vi "Constants.vi"() -> ()   [LabVIEW 2015, in "DDS Custom Device Shared.lvlib"]
doc: "Use this Global VI to access the GUIDs assigned to the page resources of the Custom Device."
uses:
  DDS Custom Device Shared.lvlib
panel:
  in  "Tab Control":enum32{"GUIDS", "Constants", "Properties"}(tab)=enum."Properties"
  in  "GUID Writer Channel":string="796baeca-3510-460a-ac62-f01a5eb8fe3f"
  in  "GUID Reader Page":string="796baeca-3510-460a-ac62-f01a5eb8fe3f"
  in  "GUID Readers Section":string="6c820a71-c73a-43d9-b216-f9ee8b776095"
  in  "GUID Writer Page":string="79fac92f-d032-46dc-bd23-f82c2cfdfdbc"
  in  "GUID Writers Section":string="dd125e97-1a18-47b4-aa06-ca880e6dc00e"
  in  "GUID DDS Custom Device":string="e2ce4079-becb-402d-aff2-142c98505f69"
  in  "Topic Cluster Bool Channel Name":string="Cluster_Bool"
  in  "Topic Cluster Sgl_Num Channel Name":string="Cluster_Sgl_Num"
  in  "Topic Sgl_Array Channel Name":string="Sgl_Array_Elem"
  in  "Topic U16_Num Channel Name":string="U16_Num"
  in  "Topic I64_Num Channel Name":string="I64_Num"
  in  "Topic I32_Num Channel Name":string="I32_Num"
  in  "Readers Section Name":string="Topic Readers"
  in  "Topic Name":string="MyTopic"
  in  "Writers Section Name":string="Topic Writers"
  in  "Channel.DataType":string="U32"
  in  "Topic.forceRead":string="forceRead"
  in  "Topic.forceExclusiveReader":string="forceExclusiveReader"
  in  "Topic.keyName":string="keyName"
  in  "Topic.forceUnboundedString":string="forceUnboundedString"
  in  "Topic.forceArrayMapping":string="forceArrayMapping"
  in  "Topic.dataWriterParticipantQoSProfile":string="dataWriterQoS"
  in  "Topic.domainParticipantQoSProfile":string="participantQoS"
  in  "Topic.typeName":string="typeName"
  in  "Topic.topicName":string="topicWriterName"
  in  "Topic.domainId":string="domainId"
  in  "Compiled.Settings":string="Compiled.Settings"
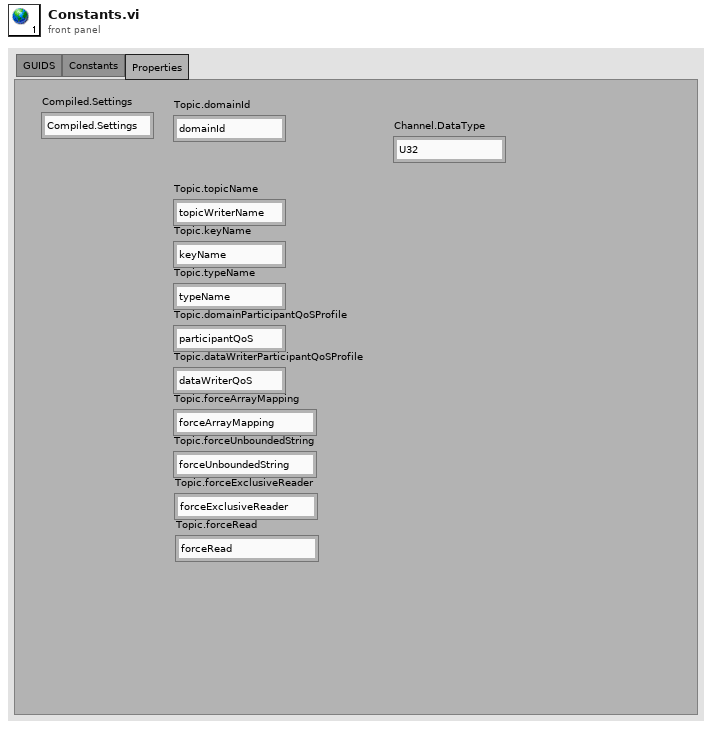
[diagram p1: front panel]
diagram:
